vi "Forward Kinematics.vi"(4 "Time step":dbl, 5 "Global acceleration in":refnum<class "Vector2.lvclass">, 6 "Acceleration in":refnum<class "Vector2.lvclass">, 7 "Velocity in":refnum<class "Vector2.lvclass">, 8 "Position in":refnum<class "Vector2.lvclass">) -> (0 "Global acceleration out":refnum<class "Vector2.lvclass">, 1 "Acceleration out":refnum<class "Vector2.lvclass">, 2 "Velocity out":refnum<class "Vector2.lvclass">, 3 "Position out":refnum<class "Vector2.lvclass">)   [LabVIEW 2022 SP3, in "PhysicsSystem.lvclass"]
uses:
  PhysicsSystem.lvclass
  PhysicsSystem.lvclass/PhysicsSystem.ctl
  Math/Vector2/Vector2.lvclass
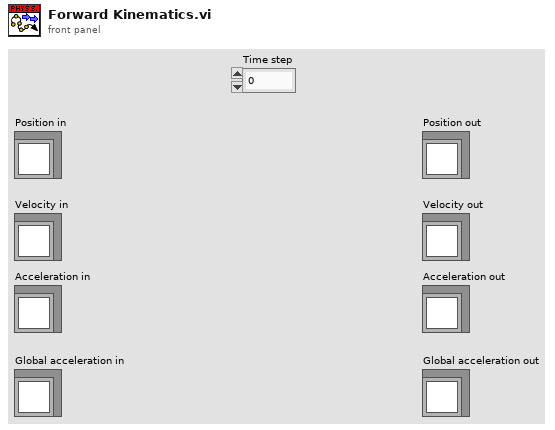
[diagram p1: front panel]
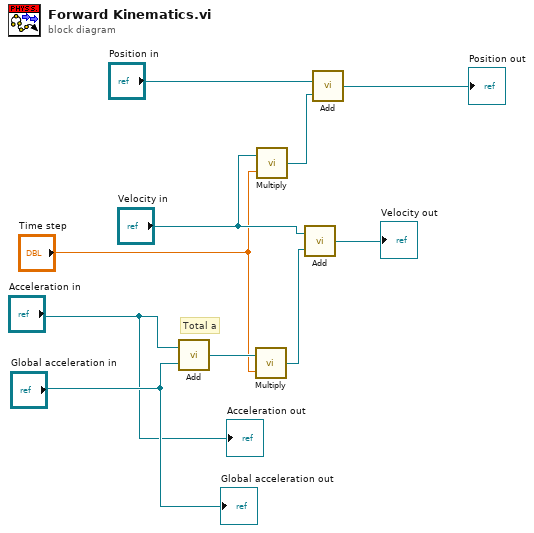
[diagram p0: block diagram]
diagram:
  # "Total a"
  n1 = call "Add.vi"("Vec2 b in"="Global acceleration in", "Vec2 a in"="Acceleration in") -> ("Vec2 out"=w10:refnum<class "Vector2.lvclass">)
  n2 = call "Multiply.vi"("Scalar"="Time step", "Vector in"=w10) -> ("Vector out"=w9:refnum<class "Vector2.lvclass">)
  n3 = call "Multiply.vi"("Scalar"="Time step", "Vector in"="Velocity in") -> ("Vector out"=w8:refnum<class "Vector2.lvclass">)
  n4 = call "Add.vi"("Vec2 b in"=w9, "Vec2 a in"="Velocity in") -> ("Vec2 out"=→"Velocity out":refnum<class "Vector2.lvclass">)
  n5 = call "Add.vi"("Vec2 b in"=w8, "Vec2 a in"="Position in") -> ("Vec2 out"=→"Position out":refnum<class "Vector2.lvclass">)
  "Acceleration out" <- "Acceleration in"
  "Global acceleration out" <- "Global acceleration in"
